vi "Is Initialized.vi"(8 "error in":errorcluster, 11 "PCAN Base Strategy in":refnum<class "PCAN Base Strategy.lvclass">) -> (0 "error out":errorcluster, 2 "Is Initialized?":bool, 3 "PCAN Base Strategy out":refnum<class "PCAN Base Strategy.lvclass">)   [LabVIEW 2024, in "PCAN Base Strategy.lvclass"]
uses:
  PCAN Base Strategy.lvclass
  PCAN Base Strategy.lvclass/PCAN Base Strategy.ctl
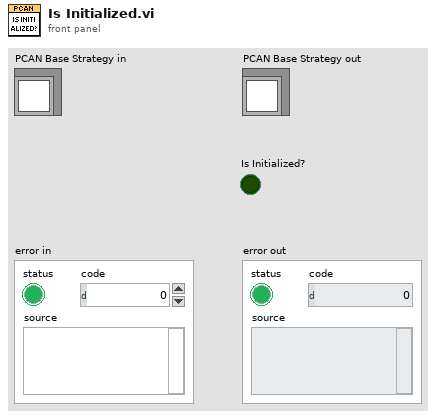
[diagram p1: front panel]
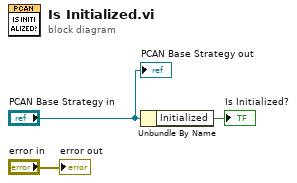
[diagram p0: block diagram]
diagram:
  n1 = Unbundle By Name("PCAN Base Strategy in") -> ("Initialized"=→"Is Initialized?":bool)
  "PCAN Base Strategy out" <- "PCAN Base Strategy in"
  "error out" <- "error in"
